vi "Rectangle2004.vi"   [LabVIEW 2013]
uses:
  <vilib>/Heliosphere Research LLC/Advanced Plotting Toolkit/api_core/NewPlotProperties.ctl
  <vilib>/Heliosphere Research LLC/Advanced Plotting Toolkit/typedefs/PlotColor.ctl
  <vilib>/Heliosphere Research LLC/Advanced Plotting Toolkit/Advanced Plotting Toolkit.lvlib
types:
  T1 = typedef "Advanced Plotting Toolkit.lvlib/NewPlotProperties.ctl" = cluster{"Background Color":T2, "Axis Background":T2, "Left Margin":dbl, "Right Margin":dbl, "Bottom Margin":dbl, "Top Margin":dbl, "Aspect Ratio":dbl}
  T2 = typedef "Advanced Plotting Toolkit.lvlib/PlotColor.ctl" = u32
  T3 = typedef "Advanced Plotting Toolkit.lvlib/PlotID.ctl" = i32
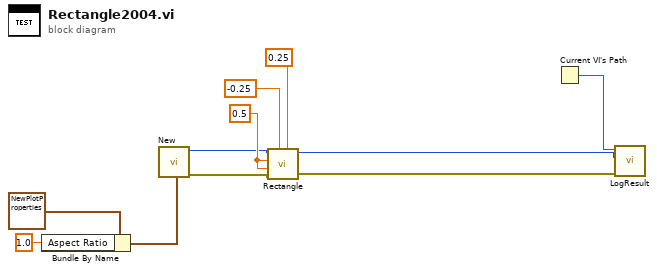
[diagram p0: block diagram]
diagram:
  w10 = 0.5 ("X Position")
  n1 = Bundle By Name(cluster=T1 {"Background Color"=2147483647, "Axis Background"=2147483647, "Left Margin"=nan, "Right Margin"=nan, "Bottom Margin"=nan, "Top Margin"=nan, "Aspect Ratio"=nan} ("New Plot Properties"), "Aspect Ratio"=1.0) -> (w4:T1)
  n2 = call <vilib>:"New.vi"("Properties"=w4) -> ("error out"=w8:errorcluster, "Plot ID"=w9:T3)  [unwired: 9 in]
  n3 = call <vilib>:"Rectangle.vi"("Height"=0.25, "Width"=-0.25 ("Radius"), "error in (no error)"=w8, "Y Position"=w10, "X Position"=w10, "Plot ID"=w9) -> ("error out"=w6:errorcluster, "Plot ID Out"=w7:T3)  [unwired: 4 in]
  n4 = Current VI's Path() -> (path=w11:path)
  n5 = call "LogResult.vi"("Test Result"=w6, "Test Artifact"=w7, "VI Path"=w11) -> ()  [unwired: 9 in]
